vi "TIFF ULS to File.vi"(8 "error in (no error)":errorcluster, 10 "refnum in":refnum<file>, 11 "TIFF in":refnum<class "TIFF ULS.lvclass">) -> (0 "error out":errorcluster, 2 "refnum out":refnum<file>)   [LabVIEW 2016, in "TIFF ULS.lvclass"]
uses:
  TIFF ULS.lvclass
  TIFF ULS.lvclass/TIFF ULS.ctl
  IFD/IFD.lvclass/IFD.ctl
  Tag/IFD_Tag.lvclass/IFD_Tag.ctl
  IFD/IFD Tag Total Size.vi
  Tag/Tag ID.vi
  Tag/Tag Data.vi
  Tag/Tag Change Value.vi
  IFD/Image Data/IFD U16 Image out.vi
  IFD/Image Data/IFD RGB Image out.vi
  IFD/Image Data/IFD SGL Image out.vi
  Tag/Tag Size.vi
  IFD/Write All Pending Data.vi
  Tag/Tag Write to File.vi
  Tag/IFD_Tag.lvclass
  IFD/IFD.lvclass
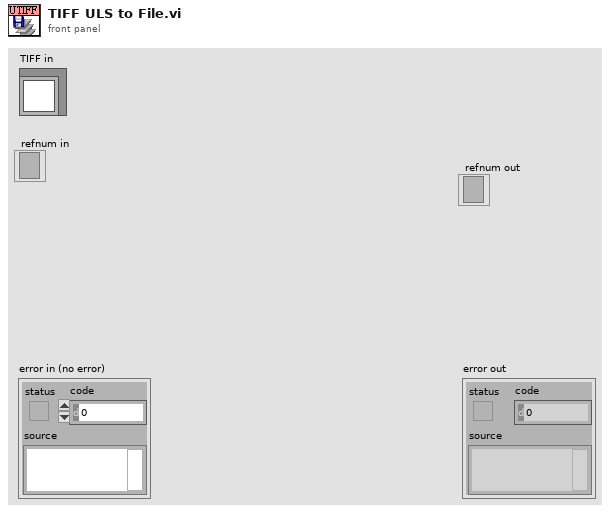
[diagram p1: front panel]
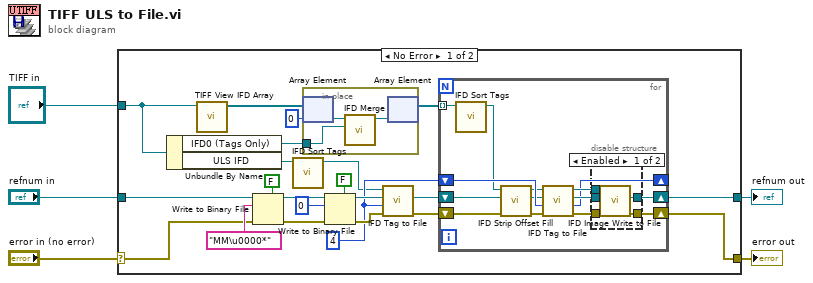
[diagram p0: block diagram]
diagram:
  n1 = case shown="No Error" "error in (no error)" {
    selector: "error in (no error)" -> [w21 w53]
    tunnel: [w12 w53] -> w4
    tunnel: "TIFF in" -> [w7 _]
    tunnel: "refnum in" -> [w11 w52]
    tunnel: [w10 w52] -> w1
    frame No Error {
      w16 = u32 4 ("Last Reference Offset")
      n2 = Unbundle By Name(w7) -> ("IFD0 (Tags Only)"=w15:refnum<class "IFD.lvclass">, "ULS IFD"=w9:refnum<class "IFD.lvclass">)
      n3 = call-dynamic "TIFF View IFD Array.vi"("TIFF in"=w7) -> ("IFD Array"=w6:refnum<class "IFD.lvclass">[])  [unwired: 9 in, 1 out]
      n4 = Write to Binary File(file (use dialog)=w11, data="MM\u0000*", error in=w21, 5:FALSE ("prepend array or string size? (T)")) -> (refnum out=w24:refnum<file>, error out=w22:errorcluster)  [unwired: 3 out]
      n5 = call "IFD Sort Tags.vi"("IFD in"=w9) -> ("IFD out"=w8:refnum<class "IFD.lvclass">)  [unwired: 9 in, 1 out]
      n6 = in-place {
        in-place-border: w15 -> [w29]
        n7 = in-place-array #1(w6, 0) -> (w30:refnum<class "IFD.lvclass">)
        n8 = call "IFD Merge.vi"("subIFD"=w29, "main IFD"=w30) -> ("IFD out"=w28:refnum<class "IFD.lvclass">)  [unwired: 8 in, 1 out]
        n9 = in-place-array #1(w28) -> (w14:refnum<class "IFD.lvclass">[])  [unwired: 1 out]
      }
      n10 = Write to Binary File(file (use dialog)=w24, data=u32 0, error in=w22, 5:FALSE ("prepend array or string size? (T)")) -> (refnum out=w19:refnum<file>, error out=w20:errorcluster)  [unwired: 3 out]
      n11 = call "IFD Tag to File.vi"("error in (no error)"=w20, "Last Reference Offset"=w16, "refnum in"=w19, "IFD in"=w8) -> ("error out"=w18:errorcluster, "refnum out"=w17:refnum<file>)  [unwired: 4 in, 2 out]
      n12 = for {
        shift-right: [w38] -> w12
        shift-left: w18 -> [w32]
        shift-right: [w40] -> w10
        shift-left: w17 -> [w34]
        shift-right: [w39] -> _
        shift-left: w16 -> [w44]
        tunnel: w14 -> [w37] mode=indexing
        n13 = call "IFD Sort Tags.vi"("IFD in"=w37) -> ("IFD out"=w36:refnum<class "IFD.lvclass">)  [unwired: 9 in, 1 out]
        n14 = call "IFD Strip Offset Fill.vi"("error in (no error)"=w32, "refnum"=w34, "IFD in"=w36) -> ("error out"=w31:errorcluster, "refnum out"=w33:refnum<file>, "IFD out"=w35:refnum<class "IFD.lvclass">)  [unwired: 6 in]
        n15 = call "IFD Tag to File.vi"("error in (no error)"=w31, "Last Reference Offset"=w44, "refnum in"=w33, "IFD in"=w35) -> ("error out"=w41:errorcluster, "Reference Offset"=w39:u32, "refnum out"=w43:refnum<file>, "IFD out"=w42:refnum<class "IFD.lvclass">)  [unwired: 4 in]
        n16 = disable-structure shown="Enabled" {
          disable-tunnel: w43 -> [w49 w51]
          disable-tunnel: w42 -> [w48 _]
          disable-tunnel: w41 -> [w47 w50]
          disable-tunnel: [w46 w51] -> w40
          disable-tunnel: [w45 w50] -> w38
          frame Enabled {
            n17 = call "IFD Image Write to File.vi"("error in (no error)"=w47, "refnum in"=w49, "IFD in"=w48) -> ("error out"=w45:errorcluster, "refnum out"=w46:refnum<file>)  [unwired: 7 in]
          }
          frame Disabled {
          }
        }
      }
    }
    frame Error {
    }
  }
  "error out" <- w4
  "refnum out" <- w1
